vi "ActiView806-Lores.vi"() -> ()   [LabVIEW 2020] (continued)
                  n1614 = call "DCviewer-Mon.vi"("N Chan In"=w4217, "Speedmode"=w4199, "Mark2"=w4201, "Channels"="Offset", "ElecGain"=w4213) -> ("First Trace"=w4218:i32, "First Half array out"=→"Offset Graph First Half":dbl[], "First Half Graph Scaling"=w4212:T36, "Second Half array out"=→"Offset Graph  Second Half":dbl[], "Second Half Graph Scaling"=w4220:T36)
                  n1615 = property on="Offset Graph First Half" class="WFGraph (strict)"() -> ("Position:Left"=w4230:i32)  [unwired: 2 in, 2 out]
                  n1616 = call "DCviewer-TP.vi"("ElecGain"=w4213, "Mark2"=w4201, "Speedmode"=w4199, "N Chan In"=w4217) -> ("Second Half array out"=→"TP Offset Graph 2":dbl[], "First Half array out"=→"TP Offset Graph 1":dbl[])
                  n1617 = Select(t=u32 16711680, s=w4228, f=u32 1970943) -> (s? t:f=w4203:u32)
                  n1618 = Unbundle(w4212) -> ("Xo"=w4222:dbl, "Xmax"=w4208:dbl, "Xmin"=w4207:dbl, "Marker values"=w4206:dbl[])
                  n1619 = Greater?(x=w4229, y=w4230) -> (0:w4231:bool)
                  n1620 = Negate(x=w4205) -> (-x=w4204:dbl)
                  n1621 = property on="Offset Graph First Half" class="WFGraph (strict)"("Plot.Fill/Pt. Color"=w4203, "X Scale.Offset and Multiplier:Offset"=w4222, "XScale.Maximum"=w4208, "XScale.Minimum"=w4207, "XScale.MarkerVals[]"=w4206) -> ()  [unwired: 2 in, 2 out]
                  n1622 = case shown="False" w4231 {
                    tunnel: w4205 -> [w4317 w4326]
                    tunnel: w4229 -> [w4318 w4325]
                    tunnel: u32 1029 ("Plot Area:Size:Width") -> [w4316 w4324]
                    tunnel: w4204 -> [w4315 w4323]
                    frame False {
                      n1623 = stacked-sequence {
                        tunnel: w4318 -> [w4320 _]
                        tunnel: w4317 -> [_ w4322]
                        tunnel: w4316 -> [w4319 _]
                        tunnel: w4315 -> [_ w4321]
                        frame #0 {
                          n1624 = property on="Offset Graph  Second Half" class="WFGraph (strict)"("Position:Left"=w4320, "Width"=w4319) -> ()  [unwired: 2 in, 2 out]
                          n1625 = property on="Offset Graph First Half" class="WFGraph (strict)"("Position:Left"=w4320, "Width"=w4319) -> ()  [unwired: 2 in, 2 out]
                        }
                        frame #1 {
                          n1626 = property on="Offset Graph First Half" class="WFGraph (strict)"("Y Scale.Range:Maximum"=w4322, "YScale.Minimum"=w4321) -> ()  [unwired: 2 in, 2 out]
                          n1627 = property on="Offset Graph  Second Half" class="WFGraph (strict)"("Y Scale.Range:Maximum"=w4322, "YScale.Minimum"=w4321) -> ()  [unwired: 2 in, 2 out]
                        }
                      }
                    }
                    frame True {
                      n1628 = stacked-sequence {
                        tunnel: w4325 -> [_ w4330]
                        tunnel: w4326 -> [w4328 _]
                        tunnel: w4324 -> [_ w4329]
                        tunnel: w4323 -> [w4327 _]
                        frame #0 {
                          n1629 = property on="Offset Graph First Half" class="WFGraph (strict)"("Y Scale.Range:Maximum"=w4328, "YScale.Minimum"=w4327) -> ()  [unwired: 2 in, 2 out]
                          n1630 = property on="Offset Graph  Second Half" class="WFGraph (strict)"("Y Scale.Range:Maximum"=w4328, "YScale.Minimum"=w4327) -> ()  [unwired: 2 in, 2 out]
                        }
                        frame #1 {
                          n1631 = property on="Offset Graph  Second Half" class="WFGraph (strict)"("Position:Left"=w4330, "Width"=w4329) -> ()  [unwired: 2 in, 2 out]
                          n1632 = property on="Offset Graph First Half" class="WFGraph (strict)"("Position:Left"=w4330, "Width"=w4329) -> ()  [unwired: 2 in, 2 out]
                        }
                      }
                    }
                  }
                  n1633 = Unbundle(w4220) -> ("Xo"=w4221:dbl, "Xmax"=w4211:dbl, "Xmin"=w4210:dbl, "Marker values"=w4209:dbl[])
                  n1634 = call "DClabels.vi"("Offset"="Offset", "Mark2"=w4201, "Speedmode"=w4199, "Mon Channels"=w4200, "Spec Labels"=w4197) -> ("DC Labels"=w4202:string[])
                  n1635 = for {
                    N: w4219 -> [_]
                    tunnel: w4202 -> [w4242]
                    tunnel: w4218 -> [w4235]
                    i -> [w4237]
                    w4245 = 0
                    w4246 = "\r"
                    n1636 = Add(x=w4235, y=w4237) -> (x+y=w4236:i32)
                    n1637 = Index Array(array=w4242, index=w4236) -> (element=w4238:string)
                    n1638 = Increment(x=w4245) -> (x+1=w4241:i32)
                    n1639 = Increment(x=w4241) -> (x+1=w4244:i32)
                    n1640 = Increment(x=w4244) -> (x+1=w4243:i32)
                    n1641 = String Subset(string=w4238, offset (0)=w4244, length (rest)=w4241) -> (substring=w4248:string)
                    n1642 = String Subset(string=w4238, offset (0)=w4245, length (rest)=w4241) -> (substring=w4250:string)
                    n1643 = String Subset(string=w4238, offset (0)=w4241, length (rest)=w4241) -> (substring=w4249:string)
                    n1644 = String Subset(string=w4238, offset (0)=w4243, length (rest)=w4241) -> (substring=w4247:string)
                    n1645 = Increment(x=w4237) -> (x+1=w4239:i32)
                    n1646 = Concatenate Strings(w4250, w4246, w4249, w4246, w4248, w4246, w4247) -> (w4240:string)
                    n1647 = case shown="64, Default" w4239 {
                      tunnel: w4240 -> [w4251 w4252 w4253 w4254 w4255 w4256 w4257 w4258 w4259 w4260 w4261 w4262 w4263 w4264 w4265 w4266 w4267 w4268 w4269 w4270 w4271 w4272 w4273 w4274 w4275 w4276 w4277 w4278 w4279 w4280 w4281 w4282 w4283 w4284 w4285 w4286 w4287 w4288 w4289 w4290 w4291 w4292 w4293 w4294 w4295 w4296 w4297 w4298 w4299 w4300 w4301 w4302 w4303 w4304 w4305 w4306 w4307 w4308 w4309 w4310 w4311 w4312 w4313 w4314]
                      frame 1 {
                        "Offset1" <- w4251
                      }
                      frame 2 {
                        "Offset2" <- w4252
                      }
                      frame 3 {
                        "Offset3" <- w4253
                      }
                      frame 4 {
                        "Offset4" <- w4254
                      }
                      frame 5 {
                        "Offset5" <- w4255
                      }
                      frame 6 {
                        "Offset6" <- w4256
                      }
                      frame 7 {
                        "Offset7" <- w4257
                      }
                      frame 8 {
                        "Offset8" <- w4258
                      }
                      frame 9 {
                        "Offset9" <- w4259
                      }
                      frame 10 {
                        "Offset10" <- w4260
                      }
                      frame 11 {
                        "Offset11" <- w4261
                      }
                      frame 12 {
                        "Offset12" <- w4262
                      }
                      frame 13 {
                        "Offset13" <- w4263
                      }
                      frame 14 {
                        "Offset14" <- w4264
                      }
                      frame 15 {
                        "Offset15" <- w4265
                      }
                      frame 16 {
                        "Offset16" <- w4266
                      }
                      frame 17 {
                        "Offset17" <- w4267
                      }
                      frame 18 {
                        "Offset18" <- w4268
                      }
                      frame 19 {
                        "Offset19" <- w4269
                      }
                      frame 20 {
                        "Offset20" <- w4270
                      }
                      frame 21 {
                        "Offset21" <- w4271
                      }
                      frame 22 {
                        "Offset22" <- w4272
                      }
                      frame 23 {
                        "Offset23" <- w4273
                      }
                      frame 24 {
                        "Offset24" <- w4274
                      }
                      frame 25 {
                        "Offset25" <- w4275
                      }
                      frame 26 {
                        "Offset26" <- w4276
                      }
                      frame 27 {
                        "Offset27" <- w4277
                      }
                      frame 28 {
                        "Offset28" <- w4278
                      }
                      frame 29 {
                        "Offset29" <- w4279
                      }
                      frame 30 {
                        "Offset30" <- w4280
                      }
                      frame 31 {
                        "Offset31" <- w4281
                      }
                      frame 32 {
                        "Offset32" <- w4282
                      }
                      frame 33 {
                        "Offset33" <- w4283
                      }
                      frame 34 {
                        "Offset34" <- w4284
                      }
                      frame 35 {
                        "Offset35" <- w4285
                      }
                      frame 36 {
                        "Offset36" <- w4286
                      }
                      frame 37 {
                        "Offset37" <- w4287
                      }
                      frame 38 {
                        "Offset38" <- w4288
                      }
                      frame 39 {
                        "Offset39" <- w4289
                      }
                      frame 40 {
                        "Offset40" <- w4290
                      }
                      frame 41 {
                        "Offset41" <- w4291
                      }
                      frame 42 {
                        "Offset42" <- w4292
                      }
                      frame 43 {
                        "Offset43" <- w4293
                      }
                      frame 44 {
                        "Offset44" <- w4294
                      }
                      frame 45 {
                        "Offset45" <- w4295
                      }
                      frame 46 {
                        "Offset46" <- w4296
                      }
                      frame 47 {
                        "Offset47" <- w4297
                      }
                      frame 48 {
                        "Offset48" <- w4298
                      }
                      frame 49 {
                        "Offset49" <- w4299
                      }
                      frame 50 {
                        "Offset50" <- w4300
                      }
                      frame 51 {
                        "Offset51" <- w4301
                      }
                      frame 52 {
                        "Offset52" <- w4302
                      }
                      frame 53 {
                        "Offset53" <- w4303
                      }
                      frame 54 {
                        "Offset54" <- w4304
                      }
                      frame 55 {
                        "Offset55" <- w4305
                      }
                      frame 56 {
                        "Offset56" <- w4306
                      }
                      frame 57 {
                        "Offset57" <- w4307
                      }
                      frame 58 {
                        "Offset58" <- w4308
                      }
                      frame 59 {
                        "Offset59" <- w4309
                      }
                      frame 60 {
                        "Offset60" <- w4310
                      }
                      frame 61 {
                        "Offset61" <- w4311
                      }
                      frame 62 {
                        "Offset62" <- w4312
                      }
                      frame 63 {
                        "Offset63" <- w4313
                      }
                      frame 64, Default {
                        "Offset64" <- w4314
                      }
                    }
                  }
                  n1648 = property on="Offset Graph  Second Half" class="WFGraph (strict)"("Plot.Fill/Pt. Color"=w4203, "X Scale.Offset and Multiplier:Offset"=w4221, "XScale.Maximum"=w4211, "XScale.Minimum"=w4210, "XScale.MarkerVals[]"=w4209) -> ()  [unwired: 2 in, 2 out]
                  n1649 = property on="TP Offset Graph 1" class="WFGraph (strict)"("YScale.Maximum"=w4205, "YScale.Minimum"=w4204, "Plot.Fill/Pt. Color"=w4203) -> ()  [unwired: 2 in, 2 out]
                  n1650 = property on="TP Offset Graph 2" class="WFGraph (strict)"("YScale.Maximum"=w4205, "YScale.Minimum"=w4204, "Plot.Fill/Pt. Color"=w4203) -> ()  [unwired: 2 in, 2 out]
                }
                frame "About ActiView", Default {
                }
              }
              n1651 = Add(x=w3354, y=w3417) -> (x+y=w3430:i32)
              n1652 = Concatenate Strings(w3370, " %" ("string")) -> (→"Jazz Batt Perc":string)
              n1653 = case shown="2" w3741 {
                tunnel: [FALSE FALSE TRUE] -> w3404
                tunnel: [i8 0 i8 2 i8 0] -> w3688
                tunnel: [FALSE TRUE FALSE] -> w3650
                frame 0, Default {
                }
                frame 1 {
                }
                frame 2 {
                }
              }
              n1654 = And(x=w3404, y="AuxReset") -> (x .and. y?=w3678:bool)
              n1655 = Or(x=w3678, y=w3681) -> (x .or. y?=w3680:bool)
              n1656 = call "Sensor.vi"("First Call"=w3431, "BreathBelt"=w3346, "Gain Cluster"=w3642, "Reset Traces"=w3680, "Sample Rate"=w3416, "Sensor Selection"="AuxFree", "8 Channel Aux Array In"=w3677) -> ("Battery Voltage"=w3548:u8, "Temperature"=→"Degrees Celcius":dbl, "Chart Array"=w3606:dbl[][], "GSR2"=→"GSR2":dbl, "GSR1"=→"GSR1":dbl)
              n1657 = Select(t=w3548, s=w3671, f=u8 0 ("t")) -> (s? t:f=→"Battery\nCapacitance" →"Battery":u8)
              n1658 = call "DeciScreen.vi"("Decimating factor"=w3401, "uV/div"=w3607, "Screen Array In"=w3606, "Max Nr of Traces"=w3550) -> ("Chart Array Out"=→"Aux Chart":dbl[][])
              n1659 = And(x=w3419, y=w3522) -> (x .and. y?=w3661:bool)
              n1660 = Unbundle By Name(w3377) -> ("Sync Errors"=w3378:i16, "Recent Sync Error"=w3374:bool)
              n1661 = Add(x="BipFree", y=w3388) -> (x+y=w3414:i32[])
              n1662 = Add(x="AnaFree", y=w3430) -> (x+y=w3410:i32[])
              n1663 = And(x="AnaReset", y=w3404) -> (x .and. y?=w3567:bool)
              n1664 = Bundle("AvgLP"="AvgLP", "AvgLPfreq"="AvgLPfreq", "AvgHP"="AvgHP", "AvgHPfreq"="AvgHPfreq") -> (w3620:T37)  [unwired: 1 out]
              n1665 = call "Ref-Avg-New.vi"("MonFreeAvg1"="MonFreeAvg1", "N Channel Array In"=w3405, "RefFreeAvg1"="RefFreeAvg1", "MonFreeAvg2"="MonFreeAvg2", "Sample Rate"=w3416, "RefFreeAvg2"="RefFreeAvg2", "Initialize Filters"=w3431, "HP Cluster"=w3620) -> ("2 Avg Chan Out"=w3610:dbl[][])
              n1666 = Not(x=w3356) -> (.not. x?=w3360:bool)
              n1667 = Less Or Equal?(x=w3357, y=u8 5) -> (x <= y?=w3359:bool)
              n1668 = Equal To 0?(x="TrigCode") -> (x = 0?=w3500:bool)
              n1669 = Compound Arithmetic op=AND(w3360, w3359, w3353) -> (w3358:bool)
              n1670 = Not Equal To 0?(x=w3354) -> (x != 0?=w3428:bool)
              n1671 = Not Equal To 0?(x=w3415) -> (x != 0?=w3382:bool)
              n1672 = Not Equal To 0?(x=w3413) -> (x != 0?=w3517:bool)
              n1673 = Array Size(array=w3610) -> (size(s)=w3627:i32[])
              n1674 = Add(x=w3378, y=w3379) -> (x+y=w3376:i16)
              "Errors:" <- w3376
              n1675 = Not Equal To 0?(x=w3379) -> (x != 0?=w3373:bool)
              n1676 = case shown="14" "Channels" {
                tunnel: [i32[] [0, 1, 2, 3, 4, 5, 6, 7, 8, 9, 10, 11, 12, 13, 14, 15, 16, 17, 18, 19, 20, 21, 22, 23, 24, 25, 26, 27, 28, 29, 30, 31, 32, 33, 34, 35, 36, 37, 38, 39, 40, 41, 42, 43, 44, 45, 46, 47, 48, 49, 50, 51, 52, 53, 54, 55, 56, 57, 58, 59, 60, 61, 62, 63, 64, 65, 66, 67, 68, 69, 70, 71, 72, 73, 74, 75, 76, 77, 78, 79, 80, 81, 82, 83, 84, 85, 86, 87, 88, 89, 90, 91, 92, 93, 94, 95, 96, 97, 98, 99, 100, 101, 102, 103, 104, 105, 106, 107, 108, 109, 110, 111, 112, 113, 114, 115, 116, 117, 118, 119, 120, 121, 122, 123, 124, 125, 126, 127, 128, 129, 130, 131, 132, 133, 134, 135, 136, 137, 138, 139, 140, 141, 142, 143, 144, 145, 146, 147, 148, 149, 150, 151, 152, 153, 154, 155, 156, 157, 158, 159, 160, 161, 162, 163, 164, 165, 166, 167, 168, 169, 170, 171, 172, 173, 174, 175, 176, 177, 178, 179, 180, 181, 182, 183, 184, 185, 186, 187, 188, 189, 190, 191, 192, 193, 194, 195, 196, 197, 198, 199, 200, 201, 202, 203, 204, 205, 206, 207, 208, 209, 210, 211, 212, 213, 214, 215, 216, 217, 218, 219, 220, 221, 222, 223, 224, 225, 226, 227, 228, 229, 230, 231, 232, 233, 234, 235, 236, 237, 238, 239, 240, 241, 242, 243, 244, 245, 246, 247, 248, 249, 250, 251, 252, 253, 254, 255, 256, 257, 258, 259, 260, 261, 262, 263] ("Array") i32[] [0, 1, 2, 3, 4, 5, 6, 7, 8, 9, 10, 11, 12, 13, 14, 15, 16, 17, 18, 19, 20, 21, 22, 23, 24, 25, 26, 27, 28, 29, 30, 31, 32, 33, 34, 35, 36, 37, 38, 39, 40, 41, 42, 43, 44, 45, 46, 47, 48, 49, 50, 51, 52, 53, 54, 55, 56, 57, 58, 59, 60, 61, 62, 63, 64, 65, 66, 67, 68, 69, 70, 71, 72, 73, 74, 75, 76, 77, 78, 79, 80, 81, 82, 83, 84, 85, 86, 87, 88, 89, 90, 91, 92, 93, 94, 95, 96, 97, 98, 99, 100, 101, 102, 103, 104, 105, 106, 107, 108, 109, 110, 111, 112, 113, 114, 115, 116, 117, 118, 119, 120, 121, 122, 123, 124, 125, 126, 127, 128, 129, 130, 131, 132, 133, 134, 135, 136, 137, 138, 139, 140, 141, 142, 143, 144, 145, 146, 147, 148, 149, 150, 151, 152, 153, 154, 155, 156, 157, 158, 159, 160, 161, 162, 163, 164, 165, 166, 167, 168, 169, 170, 171, 172, 173, 174, 175, 176, 177, 178, 179, 180, 181, 182, 183, 184, 185, 186, 187, 188, 189, 190, 191, 192, 193, 194, 195, 196, 197, 198, 199, 200, 201, 202, 203, 204, 205, 206, 207, 208, 209, 210, 211, 212, 213, 214, 215, 216, 217, 218, 219, 220, 221, 222, 223, 224, 225, 226, 227, 228, 229, 230, 231, 232, 233, 234, 235, 236, 237, 238, 239, 240, 241, 242, 243, 244, 245, 246, 247, 248, 249, 250, 251, 252, 253, 254, 255] ("All Channels") i32[] [0, 1, 2, 3, 4, 5, 6, 7, 8, 9, 10, 11, 12, 13, 14, 15, 16, 17, 18, 19, 20, 21, 22, 23, 24, 25, 26, 27, 28, 29, 30, 31, 32, 33, 34, 35, 36, 37, 38, 39, 40, 41, 42, 43, 44, 45, 46, 47, 48, 49, 50, 51, 52, 53, 54, 55, 56, 57, 58, 59, 60, 61, 62, 63, 64, 65, 66, 67, 68, 69, 70, 71, 72, 73, 74, 75, 76, 77, 78, 79, 80, 81, 82, 83, 84, 85, 86, 87, 88, 89, 90, 91, 92, 93, 94, 95, 96, 97, 98, 99, 100, 101, 102, 103, 104, 105, 106, 107, 108, 109, 110, 111, 112, 113, 114, 115, 116, 117, 118, 119, 120, 121, 122, 123, 124, 125, 126, 127, 128, 129, 130, 131, 132, 133, 134, 135, 136, 137, 138, 139, 140, 141, 142, 143, 144, 145, 146, 147, 148, 149, 150, 151, 152, 153, 154, 155, 156, 157, 158, 159] ("Array") i32[] [0, 1, 2, 3, 4, 5, 6, 7, 8, 9, 10, 11, 12, 13, 14, 15, 16, 17, 18, 19, 20, 21, 22, 23, 24, 25, 26, 27, 28, 29, 30, 31, 32, 33, 34, 35, 36, 37, 38, 39, 40, 41, 42, 43, 44, 45, 46, 47, 48, 49, 50, 51, 52, 53, 54, 55, 56, 57, 58, 59, 60, 61, 62, 63, 64, 65, 66, 67, 68, 69, 70, 71, 72, 73, 74, 75, 76, 77, 78, 79, 80, 81, 82, 83, 84, 85, 86, 87, 88, 89, 90, 91, 92, 93, 94, 95, 96, 97, 98, 99, 100, 101, 102, 103, 104, 105, 106, 107, 108, 109, 110, 111, 112, 113, 114, 115, 116, 117, 118, 119, 120, 121, 122, 123, 124, 125, 126, 127] ("Array") i32[] [0, 1, 2, 3, 4, 5, 6, 7, 8, 9, 10, 11, 12, 13, 14, 15, 16, 17, 18, 19, 20, 21, 22, 23, 24, 25, 26, 27, 28, 29, 30, 31, 32, 33, 34, 35, 36, 37, 38, 39, 40, 41, 42, 43, 44, 45, 46, 47, 48, 49, 50, 51, 52, 53, 54, 55, 56, 57, 58, 59, 60, 61, 62, 63] ("Array") i32[] [0, 1, 2, 3, 4, 5, 6, 7, 8, 9, 10, 11, 12, 13, 14, 15, 16, 17, 18, 19, 20, 21, 22, 23, 24, 25, 26, 27, 28, 29, 30, 31] ("Array") i32[] [32, 33, 34, 35, 36, 37, 38, 39, 40, 41, 42, 43, 44, 45, 46, 47, 48, 49, 50, 51, 52, 53, 54, 55, 56, 57, 58, 59, 60, 61, 62, 63] ("Array") i32[] [64, 65, 66, 67, 68, 69, 70, 71, 72, 73, 74, 75, 76, 77, 78, 79, 80, 81, 82, 83, 84, 85, 86, 87, 88, 89, 90, 91, 92, 93, 94, 95] ("Array") i32[] [96, 97, 98, 99, 100, 101, 102, 103, 104, 105, 106, 107, 108, 109, 110, 111, 112, 113, 114, 115, 116, 117, 118, 119, 120, 121, 122, 123, 124, 125, 126, 127] ("Array") i32[] [128, 129, 130, 131, 132, 133, 134, 135, 136, 137, 138, 139, 140, 141, 142, 143, 144, 145, 146, 147, 148, 149, 150, 151, 152, 153, 154, 155, 156, 157, 158, 159] ("Array") i32[] [160, 161, 162, 163, 164, 165, 166, 167, 168, 169, 170, 171, 172, 173, 174, 175, 176, 177, 178, 179, 180, 181, 182, 183, 184, 185, 186, 187, 188, 189, 190, 191] ("Array") i32[] [192, 193, 194, 195, 196, 197, 198, 199, 200, 201, 202, 203, 204, 205, 206, 207, 208, 209, 210, 211, 212, 213, 214, 215, 216, 217, 218, 219, 220, 221, 222, 223] ("Array") i32[] [224, 225, 226, 227, 228, 229, 230, 231, 232, 233, 234, 235, 236, 237, 238, 239, 240, 241, 242, 243, 244, 245, 246, 247, 248, 249, 250, 251, 252, 253, 254, 255] ("Array") w4472 w4475] -> w3389
                tunnel: [w4444 w4446 w4448 w4450 w4452 w4454 w4456 w4458 w4460 w4462 w4464 w4466 w4468 w4470 T5."Enabled" ("Disabled")] -> w3390
                tunnel: w3388 -> [_ _ _ _ _ _ _ _ _ _ _ _ _ w4471 _]
                tunnel: "MonFree" -> [_ _ _ _ _ _ _ _ _ _ _ _ _ _ w4475]
                tunnel: T5."Disabled and Grayed Out" ("Disabled") -> [w4444 w4446 w4448 w4450 w4452 w4454 w4456 w4458 w4460 w4462 w4464 w4466 w4468 w4470 _]
                frame 0, Default {
                }
                frame 1 {
                }
                frame 2 {
                }
                frame 3 {
                }
                frame 4 {
                }
                frame 5 {
                }
                frame 6 {
                }
                frame 7 {
                }
                frame 8 {
                }
                frame 9 {
                }
                frame 10 {
                }
                frame 11 {
                }
                frame 12 {
                }
                frame 13 {
                  n1677 = Add(x=i32[] [0, 1, 2, 3, 4, 5, 6, 7] ("Array"), y=w4471) -> (x+y=w4472:i32[])
                }
                frame 14 {
                }
              }
              n1678 = Add(x="JazzFree", y=w3417) -> (x+y=w3402:i32[])
              n1679 = Not(x=w3500) -> (.not. x?=w3639:bool)
              n1680 = Select(t=w3410, s=w3517, f=i32[] []) -> (s? t:f=w3518:i32[])
              n1681 = And(x="JazzReset", y=w3404) -> (x .and. y?=w3423:bool)
              n1682 = Select(t=w3402, s=w3428, f=i32[] []) -> (s? t:f=w3424:i32[])
              n1683 = Index Array(array=w3627) -> (element=w3622:i32)  [unwired: 1 in]
              n1684 = case shown="True" w3631 {
                selector: w3631 -> [_ w3951]
                tunnel: w3636 -> [w3948 _]
                tunnel: w3637 -> [w3949 _]
                tunnel: [w3949 w3962] -> w3400
                tunnel: [w3948 w3962] -> w3399
                tunnel: w3622 -> [_ w3961]
                tunnel: w3629 -> [w3947 w3950]
                tunnel: [w3947 w3960] -> w3630
                tunnel: w3459 -> [_ w3955]
                frame False {
                }
                frame True {
                  w3952 = 0 ("Rejected Sweeps")
                  # "Initilaize Buffers"
                  n1685 = Multiply(x="AvgSweep", y=w3955) -> (x*y=w3959:i32)
                  n1686 = To Double Precision Float(number=w3959) -> (double precision float=w3958:dbl)
                  n1687 = Divide(x=w3958, y=1000.0) -> (x/y=w3956:dbl)
                  n1688 = To Long Integer(number=w3956) -> (32bit integer=w3953:i32)
                  n1689 = local write "Valid Sweeps"(w3952) -> ()
                  n1690 = Bundle By Name(cluster=w3950, "Start Averaging"=w3951, "Busy Averaging"=w3951, "Sweep Lenght in Samples"=w3953, "Valid Sweeps"=w3952, "Rejected Sweeps"=w3952, "First Graph Update"=w3951) -> (w3960:T11)
                  n1691 = Initialize Array(0.0 ("element"), w3961, w3953) -> (w3962:dbl[][])
                  n1692 = local write "Rejected Sweeps"(w3952) -> ()
                }
              }
              n1693 = Select(t=w3414, s=w3382, f=i32[] []) -> (s? t:f=w3525:i32[])
              n1694 = And(x=w3374, y=w3373) -> (x .and. y?=w3453:bool)
              n1695 = property on="Trigger Code" class="Pict"("Visible"=w3639) -> ()  [unwired: 2 in, 2 out]
              n1696 = call "Ref-Jazz1.vi"("Initialize Filters"=w3425, "Center Traces"=w3423, "Channels"=w3424, "Channel Array In"=w3405) -> ("Screen signals Out"=w3447:dbl[][])  [unwired: 4 out]
              n1697 = property on="Trigger Chart" class="WFChart (strict)"("Visible"=w3500) -> ()  [unwired: 2 in, 2 out]
              n1698 = Select(t=T5."Disabled and Grayed Out" ("Disabled"), s=w3403, f=T5."Enabled" ("Disabled")) -> (s? t:f=w3418:T5)
              n1699 = Array Size(array=w3424) -> (size(s)=w3437:i32)
              n1700 = case shown="True" "AddTP" {
                tunnel: w3389 -> [w3755 w3757]
                tunnel: [w3755 w3756] -> w3387
                tunnel: w3388 -> [_ w3759]
                frame False {
                }
                frame True {
                  n1701 = Add(x=i32[] [0, 1, 2, 3, 4, 5, 6, 7] ("Array"), y=w3759) -> (x+y=w3758:i32[])
                  n1702 = Build Array (concatenate)(w3757, w3758) -> (w3756:i32[])
                }
              }
              n1703 = Array Size(array=w3442) -> (size(s)=w3444:i32)
              n1704 = property on="JazzFree" class="LstBox (strict)"("Disabled"=w3418) -> ()  [unwired: 2 in, 2 out]
              n1705 = Not Equal?(x=w3437, y=w3444) -> (x != y?=w3432:bool)
              n1706 = Not Equal?(x=w3424, y=w3442) -> (x != y?=w3443:bool[])
              n1707 = property on="Dummy String" class="Str"("Visible"=w3500) -> ()  [unwired: 2 in, 2 out]
              n1708 = Bundle("MonLP"="MonLP", "MonLPfreq"="MonLPfreq", "MonHP"="MonHP", "MonHPfreq"="MonHPfreq") -> (w3719:T38)  [unwired: 1 out]
              n1709 = Or Array Elements(Boolean array=w3443) -> (logical OR=w3434:bool)
              n1710 = Bundle("BipLP"="BipLP", "BipLPfreq"="BipLPfreq", "BipHP"="BipHP", "BipHPfreq"="BipHPfreq") -> (w3597:T39)  [unwired: 1 out]
              n1711 = call "Ref-Bip-New.vi"("Channel Array In"=w3405, "Channels"=w3525, "Center Traces"=w3404, "Initialize Filter"=w3683, "Sample Rate"=w3416, "Filter Cluster"=w3597, "ElecGain"=w3348) -> ("Screen signals Out"=w3682:dbl[][])
              n1712 = Bundle By Name(cluster=w3377, "Sync Errors"=w3376, "Recent Sync Error"=w3373) -> (w3375:T27)
              n1713 = Bundle("AnaLP"="AnaLP", "AnaLPfreq"="AnaLPfreq", "AnaHP"="AnaHP", "AnaHPfreq"="AnaHPfreq") -> (w3647:T40)  [unwired: 1 out]
              n1714 = call "Ref-Ana.vi"("Channel Array In"=w3405, "Channels"=w3518, "Center Traces"=w3567, "Initialize Filters"=w3568, "Sample Rate"=w3416, "Filter Cluster"=w3647) -> ("Screen signals Out"=w3649:dbl[][])  [unwired: 1 out]
              n1715 = call "DeciScreen.vi"("Decimating factor"=w3401, "uV/div"=w3426, "Screen Array In"=w3447, "Max Nr of Traces"=w3354) -> ("Chart Array Out"=→"Jazz Chart":dbl[][])
              n1716 = Equal?(x=T2."Analog Input Box" ("Charts/Graphs"), y="Charts/Graphs") -> (x = y?=w3644:bool)
              n1717 = Compound Arithmetic op=OR(w3434, w3432, w3431) -> (w3433:bool)
              n1718 = Array Subset(array=w3387, length=w3381) -> (w3386:i32[])  [unwired: 1 in]
              n1719 = Bundle("Speed Mode"=w3327, "Save Subset"=w3523, w3386, "Add Touchproofs"=w3527, "Mon Channels"=w3388, "Bip Channels"=w3415, "Add Sensors"=w3420, w3411, "Add Jazz"=w3421, w3402, "Add Anas"=w3429, w3410, "Save Box"=w3409) -> (w3529:T41)  [unwired: 1 out]
              n1720 = call "Act_Save_Daisy.vi"("Save Selection Cluster"=w3529, "Status Channel  In"=w3406, "Data In"=w3412, "Samples per Record"=w3459, "BDF Buffer In"=w3458, "Index in Byte In"=w3457) -> ("Nr of Chan Saved"=w3611:i32, "BDF Buffer Out"=w3698:u8[], "Index in Byte Out"=w3699:i32)
              n1721 = Decrement(x=w3611) -> (x-1=w3618:i32)
              n1722 = Format Into String(format string="%d" ("Format String"), w3618) -> (resulting string=w3616:string)  [unwired: 2 in, 1 out]
              n1723 = Concatenate Strings(w3616, " + 1" ("Substring")) -> (w3614:string)
              n1724 = Select(t=w3614, s=w3419, f="0 + 0") -> (s? t:f=→"Nr Chan Saved":string)
              n1725 = Select(t=w3332, s=w3661, f=w3390) -> (s? t:f=w3708:T5)
              n1726 = Select(t=w3332, s=w3661, f=T5."Enabled" ("Disabled")) -> (s? t:f=w3384:T5)
              n1727 = property on="MonFree" class="LstBox (strict)"("Disabled"=w3708) -> ()  [unwired: 2 in, 2 out]
              n1728 = Select(t=w3384, s=w3382, f=w3332) -> (s? t:f=w3383:T5)
              n1729 = property on="Channels" class="Ring (strict)"("Disabled"=w3384) -> ()  [unwired: 2 in, 2 out]
              n1730 = property on="AddTP" class="Bool (strict)"("Disabled"=w3383) -> ()  [unwired: 2 in, 2 out]
              n1731 = case shown="True" w3644 {
                tunnel: w3405 -> [_ w3968]
                tunnel: w3430 -> [_ w3966]
                frame False {
                }
                frame True {
                  n1732 = Add(x=w3966, y="AnaOffset") -> (x+y=w3964:i32)
                  n1733 = call "DCviewer-Ana.vi"("Ana Channels"=w3964, "N Chan In"=w3968) -> ("1 Chan array out"=→"Ana Offset Graph":dbl[])
                }
              }
              n1734 = Unbundle By Name(w3733) -> ("End of Screen"=w3669:bool, "Prop Screen Minimum"=w3665:i64, "Screen Position"=w3504:i32)
              n1735 = call "TriggerScreen.vi"("Screen Position"=w3504, "Downsample Correction"=w3449, "Block Cluster"=w3499, "[user-specified font]"=T13 {"Font Name:"="Microsoft Sans Serif", "Size"=12, "Strikeout?"=FALSE, "Italic?"=FALSE, "Underline?"=FALSE, "Outline?"=FALSE, "Shadow?"=FALSE, "Bold?"=FALSE}, "Old picture 2"=w3407, "Old picture 1"=w3408, "Status Channel  In"=w3406, "TrigCode"="TrigCode") -> ("New picture 2"=w3502:picture, "New picture 1"=w3503:picture)
              n1736 = case shown="\"Auxiliary Sensors\"" "Charts/Graphs" {
                tunnel: [T1."Monopolar" ("Left Sidebar") T1."Bipolar" ("Left Sidebar") T1."Offset" ("Left Sidebar") T1."Average" ("Left Sidebar") T1."Sensors" ("Left Sidebar") T1."Jazz" ("Left Sidebar") T1."Analog" ("Left Sidebar") T1."Initialization" ("Left Sidebar")] -> w3452
                frame "Monopolar Display" {
                }
                frame "Bipolar Leads" {
                }
                frame "Electrode Offset" {
                }
                frame "Event Related Average" {
                }
                frame "Auxiliary Sensors" {
                }
                frame "Jazz Eyetracker" {
                }
                frame "Analog Input Box" {
                }
                frame "About ActiView", Default {
                }
              }
              "Left Sidebar" <- w3452
              n1737 = Select(t=w3503, s=w3542, f=w3502) -> (s? t:f=→"Trigger Code":picture)
              n1738 = case shown="15" "MonScale" {
                tunnel: [5.0 10.0 20.0 50.0 100.0 200.0 500.0 1000.0 2000.0 5000.0 10000.0 20000.0 50000.0 100000.0 200000.0 500000.0] -> w3711
                frame 0, Default {
                }
                frame 1 {
                }
                frame 2 {
                }
                frame 3 {
                }
                frame 4 {
                }
                frame 5 {
                }
                frame 6 {
                }
                frame 7 {
                }
                frame 8 {
                }
                frame 9 {
                }
                frame 10 {
                }
                frame 11 {
                }
                frame 12 {
                }
                frame 13 {
                }
                frame 14 {
                }
                frame 15 {
                }
              }
              n1739 = case shown="18" "AnaScale" {
                tunnel: [5.0 10.0 20.0 50.0 100.0 200.0 500.0 1000.0 2000.0 5000.0 10000.0 20000.0 50000.0 100000.0 200000.0 500000.0 1000000.0 2000000.0 4000000.0] -> w3658
                frame 0, Default {
                }
                frame 1 {
                }
                frame 2 {
                }
                frame 3 {
                }
                frame 4 {
                }
                frame 5 {
                }
                frame 6 {
                }
                frame 7 {
                }
                frame 8 {
                }
                frame 9 {
                }
                frame 10 {
                }
                frame 11 {
                }
                frame 12 {
                }
                frame 13 {
                }
                frame 14 {
                }
                frame 15 {
                }
                frame 16 {
                }
                frame 17 {
                }
                frame 18 {
                }
              }
              n1740 = case shown="15" "BipScale" {
                tunnel: [5.0 10.0 20.0 50.0 100.0 200.0 500.0 1000.0 2000.0 5000.0 10000.0 20000.0 50000.0 100000.0 200000.0 500000.0] -> w3700
                frame 0, Default {
                }
                frame 1 {
                }
                frame 2 {
                }
                frame 3 {
                }
                frame 4 {
                }
                frame 5 {
                }
                frame 6 {
                }
                frame 7 {
                }
                frame 8 {
                }
                frame 9 {
                }
                frame 10 {
                }
                frame 11 {
                }
                frame 12 {
                }
                frame 13 {
                }
                frame 14 {
                }
                frame 15 {
                }
              }
              n1741 = Build Array(w3456, w3455, w3453, w3456, w3356, w3355) -> (w3663:bool[])
              n1742 = Compound Arithmetic op=OR(w3455, w3453, w3356, w3355) -> (w3454:bool)
              n1743 = Array Size(array=w3386) -> (size(s)=w3495:i32)
              n1744 = Array Size(array=w3715) -> (size(s)=w3730:i32)
              n1745 = case shown="True" w3433 {
                tunnel: w3437 -> [_ w3766]
                tunnel: w3424 -> [_ w3763]
                tunnel: w3448 -> [_ w3761]
                frame False {
                }
                frame True {
                  w3764 = 9  # Nr of Jazz Labels
                  w3771 = -292.0  # Upper Y-value
                  w3773 = 532.0  # Lower Y-value
                  n1746 = Not Equal To 0?(x=w3766) -> (x != 0?=w3767:bool)
                  n1747 = Increment(x=w3766) -> (x+1=w3768:i32)
                  n1748 = Subtract(x=w3773, y=w3771) -> (x-y=w3772:dbl)
                  n1749 = Select(t=w3768, s=w3767, f=2) -> (s? t:f=w3762:i32)
                  n1750 = To Double Precision Float(number=w3762) -> (double precision float=w3765:dbl)
                  n1751 = Divide(x=w3772, y=w3765) -> (x/y=w3770:dbl)
                  n1752 = for {
                    N: w3764 -> [_]
                    tunnel: w3761 -> [w3782]
                    tunnel: w3763 -> [w3779]
                    tunnel: w3771 -> [w3784]
                    tunnel: w3770 -> [w3783]
                    tunnel: w3766 -> [w3780]
                    i -> [w3775]
                    n1753 = Greater?(x=w3780, y=w3775) -> (0:w3781:bool)
                    n1754 = Increment(x=w3775) -> (x+1=w3778:i32)
                    n1755 = case shown="True" w3781 {
                      tunnel: w3784 -> [_ w3816]
                      tunnel: w3783 -> [_ w3815]
                      tunnel: w3782 -> [_ w3806]
                      tunnel: w3778 -> [_ w3811]
                      tunnel: ["" w3807] -> w3777
                      tunnel: [0 w3810] -> w3776
                      tunnel: w3779 -> [_ w3809]
                      tunnel: w3775 -> [_ w3808]
                      frame False {
                      }
                      frame True {
                        n1756 = Index Array(array=w3809, index=w3808) -> (element=w3805:i32)
                        n1757 = To Double Precision Float(number=w3811) -> (double precision float=w3814:dbl)
                        n1758 = Index Array(array=w3806, index=w3805) -> (element=w3812:string)
                        n1759 = Multiply(x=w3815, y=w3814) -> (x*y=w3817:dbl)
                        n1760 = Add(x=w3816, y=w3817) -> (x+y=w3818:dbl)
                        n1761 = String Subset(string=w3812, length (rest)=4 ("length (rest)")) -> (substring=w3807:string)  [unwired: 1 out]
                        n1762 = To Long Integer(number=w3818) -> (32bit integer=w3810:i32)
                      }
                    }
                    n1763 = case shown="9, Default" w3778 {
                      tunnel: w3777 -> [w3786 w3788 w3790 w3792 w3794 w3796 w3798 w3800 w3802]
                      tunnel: w3776 -> [w3785 w3787 w3789 w3791 w3793 w3795 w3797 w3799 w3801]
                      frame 1 {
                        n1764 = property on="Jazz1" class="Str"("Top"=w3785) -> ()  [unwired: 2 in, 2 out]
                        "Jazz1" <- w3786
                      }
                      frame 2 {
                        n1765 = property on="Jazz2" class="Str"("Top"=w3787) -> ()  [unwired: 2 in, 2 out]
                        "Jazz2" <- w3788
                      }
                      frame 3 {
                        n1766 = property on="Jazz3" class="Str"("Top"=w3789) -> ()  [unwired: 2 in, 2 out]
                        "Jazz3" <- w3790
                      }
                      frame 4 {
                        n1767 = property on="Jazz4" class="Str"("Top"=w3791) -> ()  [unwired: 2 in, 2 out]
                        "Jazz4" <- w3792
                      }
                      frame 5 {
                        n1768 = property on="Jazz5" class="Str"("Top"=w3793) -> ()  [unwired: 2 in, 2 out]
                        "Jazz5" <- w3794
                      }
                      frame 6 {
                        n1769 = property on="Jazz6" class="Str"("Top"=w3795) -> ()  [unwired: 2 in, 2 out]
                        "Jazz6" <- w3796
                      }
                      frame 7 {
                        n1770 = property on="Jazz7" class="Str"("Top"=w3797) -> ()  [unwired: 2 in, 2 out]
                        "Jazz7" <- w3798
                      }
                      frame 8 {
                        n1771 = property on="Jazz8" class="Str"("Top"=w3799) -> ()  [unwired: 2 in, 2 out]
                        "Jazz8" <- w3800
                      }
                      frame 9, Default {
                        n1772 = property on="Jazz9" class="Str"("Top"=w3801) -> ()  [unwired: 2 in, 2 out]
                        "Jazz9" <- w3802
                      }
                    }
                  }
                  n1773 = To Double Precision Float(number=w3762) -> (double precision float=w3774:dbl)
                  n1774 = property on="Jazz Chart" class="WFChart (strict)"("YScale.Maximum"=w3774) -> ()  [unwired: 2 in, 2 out]
                }
              }
              n1775 = Boolean Array To Number(Boolean array=w3663) -> (number=w3372:u32)
              n1776 = Bundle("AvgAbsReject"="AvgAbsReject", "AvgRelReject"="AvgRelReject") -> (w3396:cluster{"AvgAbsReject":dbl, "AvgRelReject":dbl})  [unwired: 1 out]
              n1777 = case shown="True" w3628 {
                selector: w3628 -> [w3934 _]
                tunnel: w3630 -> [w3933 w3938]
                tunnel: w3610 -> [_ w3946]
                tunnel: [w3932 w3937] -> w3633
                tunnel: [w3931 w3941] -> w3635
                tunnel: "AvgTrigLog" -> [_ w3945]
                tunnel: "AvgTrigSel" -> [_ w3944]
                tunnel: w3400 -> [w3931 w3943]
                tunnel: w3399 -> [w3930 w3942]
                tunnel: [w3930 w3940] -> w3398
                tunnel: w3351 -> [_ w3939]
                tunnel: w3396 -> [_ w3936]
                tunnel: [T16 {"Sweeping"=FALSE, "RejAbs"=FALSE, "RejDif"=FALSE} ("Sweep/Reject Cluster Out") w3935] -> w3394
                frame False {
                  n1778 = Bundle By Name(cluster=w3933, "Busy Averaging"=w3934) -> (w3932:T11)
                }
                frame True {
                  n1779 = call "Avg-Sweep-Rev.vi"("Triggers Boolean"=w3939, "Reject Cluster In"=w3936, "AvgTrigLog"=w3945, "AvgTrigSel"=w3944, "Noise Total"=w3942, "Average Total"=w3943, "Processed signals In"=w3946, "Avg Cluster In"=w3938) -> ("Noise Total Out"=w3940:dbl[][], "Average Total Out"=w3941:dbl[][], "Avg Cluster Out"=w3937:T11, "Sweep/Reject Cluster Out"=w3935:T16)
                }
              }
              n1780 = Not Equal?(x=w3495, y=w3730) -> (x != y?=w3693:bool)
              n1781 = Not Equal?(x=w3386, y=w3715) -> (x != y?=w3729:bool[])
              n1782 = case shown="8" "Reference" {
                tunnel: [i32[] [] i32[] [0, 1, 2, 3, 4, 5, 6, 7, 8, 9, 10, 11, 12, 13, 14, 15, 16, 17, 18, 19, 20, 21, 22, 23, 24, 25, 26, 27, 28, 29, 30, 31, 32, 33, 34, 35, 36, 37, 38, 39, 40, 41, 42, 43, 44, 45, 46, 47, 48, 49, 50, 51, 52, 53, 54, 55, 56, 57, 58, 59, 60, 61, 62, 63, 64, 65, 66, 67, 68, 69, 70, 71, 72, 73, 74, 75, 76, 77, 78, 79, 80, 81, 82, 83, 84, 85, 86, 87, 88, 89, 90, 91, 92, 93, 94, 95, 96, 97, 98, 99, 100, 101, 102, 103, 104, 105, 106, 107, 108, 109, 110, 111, 112, 113, 114, 115, 116, 117, 118, 119, 120, 121, 122, 123, 124, 125, 126, 127, 128, 129, 130, 131, 132, 133, 134, 135, 136, 137, 138, 139, 140, 141, 142, 143, 144, 145, 146, 147, 148, 149, 150, 151, 152, 153, 154, 155, 156, 157, 158, 159, 160, 161, 162, 163, 164, 165, 166, 167, 168, 169, 170, 171, 172, 173, 174, 175, 176, 177, 178, 179, 180, 181, 182, 183, 184, 185, 186, 187, 188, 189, 190, 191, 192, 193, 194, 195, 196, 197, 198, 199, 200, 201, 202, 203, 204, 205, 206, 207, 208, 209, 210, 211, 212, 213, 214, 215, 216, 217, 218, 219, 220, 221, 222, 223, 224, 225, 226, 227, 228, 229, 230, 231, 232, 233, 234, 235, 236, 237, 238, 239, 240, 241, 242, 243, 244, 245, 246, 247, 248, 249, 250, 251, 252, 253, 254, 255, 256, 257, 258, 259, 260, 261, 262, 263] ("Array") i32[] [0, 1, 2, 3, 4, 5, 6, 7, 8, 9, 10, 11, 12, 13, 14, 15, 16, 17, 18, 19, 20, 21, 22, 23, 24, 25, 26, 27, 28, 29, 30, 31, 32, 33, 34, 35, 36, 37, 38, 39, 40, 41, 42, 43, 44, 45, 46, 47, 48, 49, 50, 51, 52, 53, 54, 55, 56, 57, 58, 59, 60, 61, 62, 63, 64, 65, 66, 67, 68, 69, 70, 71, 72, 73, 74, 75, 76, 77, 78, 79, 80, 81, 82, 83, 84, 85, 86, 87, 88, 89, 90, 91, 92, 93, 94, 95, 96, 97, 98, 99, 100, 101, 102, 103, 104, 105, 106, 107, 108, 109, 110, 111, 112, 113, 114, 115, 116, 117, 118, 119, 120, 121, 122, 123, 124, 125, 126, 127, 128, 129, 130, 131, 132, 133, 134, 135, 136, 137, 138, 139, 140, 141, 142, 143, 144, 145, 146, 147, 148, 149, 150, 151, 152, 153, 154, 155, 156, 157, 158, 159, 160, 161, 162, 163, 164, 165, 166, 167, 168, 169, 170, 171, 172, 173, 174, 175, 176, 177, 178, 179, 180, 181, 182, 183, 184, 185, 186, 187, 188, 189, 190, 191, 192, 193, 194, 195, 196, 197, 198, 199, 200, 201, 202, 203, 204, 205, 206, 207, 208, 209, 210, 211, 212, 213, 214, 215, 216, 217, 218, 219, 220, 221, 222, 223, 224, 225, 226, 227, 228, 229, 230, 231, 232, 233, 234, 235, 236, 237, 238, 239, 240, 241, 242, 243, 244, 245, 246, 247, 248, 249, 250, 251, 252, 253, 254, 255] ("All Channels") i32[] [0, 1, 2, 3, 4, 5, 6, 7, 8, 9, 10, 11, 12, 13, 14, 15, 16, 17, 18, 19, 20, 21, 22, 23, 24, 25, 26, 27, 28, 29, 30, 31, 32, 33, 34, 35, 36, 37, 38, 39, 40, 41, 42, 43, 44, 45, 46, 47, 48, 49, 50, 51, 52, 53, 54, 55, 56, 57, 58, 59, 60, 61, 62, 63, 64, 65, 66, 67, 68, 69, 70, 71, 72, 73, 74, 75, 76, 77, 78, 79, 80, 81, 82, 83, 84, 85, 86, 87, 88, 89, 90, 91, 92, 93, 94, 95, 96, 97, 98, 99, 100, 101, 102, 103, 104, 105, 106, 107, 108, 109, 110, 111, 112, 113, 114, 115, 116, 117, 118, 119, 120, 121, 122, 123, 124, 125, 126, 127, 128, 129, 130, 131, 132, 133, 134, 135, 136, 137, 138, 139, 140, 141, 142, 143, 144, 145, 146, 147, 148, 149, 150, 151, 152, 153, 154, 155, 156, 157, 158, 159] ("Array") i32[] [0, 1, 2, 3, 4, 5, 6, 7, 8, 9, 10, 11, 12, 13, 14, 15, 16, 17, 18, 19, 20, 21, 22, 23, 24, 25, 26, 27, 28, 29, 30, 31, 32, 33, 34, 35, 36, 37, 38, 39, 40, 41, 42, 43, 44, 45, 46, 47, 48, 49, 50, 51, 52, 53, 54, 55, 56, 57, 58, 59, 60, 61, 62, 63, 64, 65, 66, 67, 68, 69, 70, 71, 72, 73, 74, 75, 76, 77, 78, 79, 80, 81, 82, 83, 84, 85, 86, 87, 88, 89, 90, 91, 92, 93, 94, 95, 96, 97, 98, 99, 100, 101, 102, 103, 104, 105, 106, 107, 108, 109, 110, 111, 112, 113, 114, 115, 116, 117, 118, 119, 120, 121, 122, 123, 124, 125, 126, 127] ("Array") i32[] [0, 1, 2, 3, 4, 5, 6, 7, 8, 9, 10, 11, 12, 13, 14, 15, 16, 17, 18, 19, 20, 21, 22, 23, 24, 25, 26, 27, 28, 29, 30, 31, 32, 33, 34, 35, 36, 37, 38, 39, 40, 41, 42, 43, 44, 45, 46, 47, 48, 49, 50, 51, 52, 53, 54, 55, 56, 57, 58, 59, 60, 61, 62, 63] ("Array") i32[] [0, 1, 2, 3, 4, 5, 6, 7, 8, 9, 10, 11, 12, 13, 14, 15, 16, 17, 18, 19, 20, 21, 22, 23, 24, 25, 26, 27, 28, 29, 30, 31] ("Array") w4441 "RefFree"] -> w3660
                tunnel: [w4426 w4428 w4430 w4432 w4434 w4436 w4438 w4440 T5."Enabled" ("Disabled")] -> w3726
                tunnel: w3386 -> [_ _ _ _ _ _ _ w4441 _]
                tunnel: w3332 -> [w4426 w4428 w4430 w4432 w4434 w4436 w4438 w4440 _]
                frame 0, Default {
                }
                frame 1 {
                }
                frame 2 {
                }
                frame 3 {
                }
                frame 4 {
                }
                frame 5 {
                }
                frame 6 {
                }
                frame 7 {
                }
                frame 8 {
                }
              }
              n1783 = call "Ref-Mon-Jazz.vi"("ElecGain"=w3348, "Reference"=w3660, "Filter Cluster"=w3719, "Sample Rate"=w3416, "Initialize Filters"=w3720, "Center Traces"=w3404, "Channel Selection"=w3386, "N Channel Array In"=w3405) -> ("Screen signals Out"=w3710:dbl[][])
              n1784 = call "DeciScreen.vi"("Decimating factor"=w3401, "uV/div"=w3711, "Screen Array In"=w3710, "Max Nr of Traces"=w3381) -> ("Chart Array Out"=→"Mon Chart":dbl[][])
              n1785 = Select(t=T5."Disabled and Grayed Out" ("Disabled"), s=w3468, f=T5."Enabled" ("Disabled")) -> (s? t:f=w3643:T5)
              n1786 = Or Array Elements(Boolean array=w3729) -> (logical OR=w3694:bool)
              n1787 = call "DeciScreen.vi"("Decimating factor"=w3401, "uV/div"=w3700, "Screen Array In"=w3682, "Max Nr of Traces"=w3415) -> ("Chart Array Out"=→"Bip Chart":dbl[][])
              n1788 = call "DeciScreen.vi"("Decimating factor"=w3401, "uV/div"=w3658, "Screen Array In"=w3649, "Max Nr of Traces"=w3413) -> ("Chart Array Out"=→"Ana Chart":dbl[][])
              n1789 = property on="AnaFree" class="LstBox (strict)"("Disabled"=w3643) -> ()  [unwired: 2 in, 2 out]
              n1790 = Compound Arithmetic op=OR(w3694, w3693, w3431) -> (w3692:bool)
              n1791 = case shown="True" w3692 {
                tunnel: w3495 -> [_ w4498]
                tunnel: w3448 -> [_ w4503]
                tunnel: w3386 -> [_ w4501]
                frame False {
                }
                frame True {
                  w4496 = -292.0  # Upper Y-value
                  w4497 = 532.0  # Lower Y-value
                  w4500 = 64  # Nr of Mon Labels
                  n1792 = Increment(x=w4498) -> (x+1=w4493:i32)
                  n1793 = Increment(x=w4500) -> (x+1=w4499:i32)
                  n1794 = Quotient & Remainder(x=w4498, y=w4499) -> (floor(x/y)=w4495:i32)  [unwired: 1 out]
                  n1795 = To Double Precision Float(number=w4493) -> (double precision float=w4502:dbl)
                  n1796 = Equal To 0?(x=w4495) -> (x = 0?=w4494:bool)
                  n1797 = property on="Mon Chart" class="WFChart (strict)"("YScale.Maximum"=w4502) -> ()  [unwired: 2 in, 2 out]
                  n1798 = for {
                    N: w4500 -> [_]
                    tunnel: w4503 -> [w4512]
                    tunnel: w4501 -> [w4513]
                    tunnel: w4498 -> [w4510]
                    tunnel: w4495 -> [w4505]
                    tunnel: w4493 -> [w4508]
                    tunnel: w4497 -> [w4507]
                    tunnel: w4496 -> [w4506]
                    tunnel: w4494 -> [w4504]
                    i -> [w4511]
                    n1799 = Increment(x=w4511) -> (x+1=w4509:i32)
                    n1800 = case shown="True" w4504 {
                      tunnel: [w4533 w4566] -> w4515
                      tunnel: [w4532 w4565] -> w4514
                      tunnel: w4509 -> [w4531 w4564]
                      tunnel: w4513 -> [w4534 w4563]
                      tunnel: w4511 -> [w4528 w4559]
                      tunnel: w4512 -> [w4535 w4562]
                      tunnel: w4510 -> [w4520 w4560]
                      tunnel: w4508 -> [_ w4555]
                      tunnel: w4507 -> [w4521 w4554]
                      tunnel: w4506 -> [w4522 w4553]
                      tunnel: w4505 -> [w4516 _]
                      frame False {
                        n1801 = Increment(x=w4516) -> (x+1=w4519:i32)
                        n1802 = To Double Precision Float(number=w4519) -> (double precision float=w4524:dbl)
                        n1803 = Increment(x=w4520) -> (x+1=w4523:i32)
                        n1804 = To Double Precision Float(number=w4523) -> (double precision float=w4525:dbl)
                        n1805 = Divide(x=w4525, y=w4524) -> (x/y=w4526:dbl)
                        n1806 = Subtract(x=w4521, y=w4522) -> (x-y=w4530:dbl)
                        n1807 = Multiply(x=w4519, y=w4528) -> (x*y=w4518:i32)
                        n1808 = Quotient & Remainder(x=w4520, y=w4519) -> (floor(x/y)=w4527:i32)  [unwired: 1 out]
                        n1809 = Divide(x=w4530, y=w4526) -> (x/y=w4529:dbl)
                        n1810 = Add(x=w4518, y=w4516) -> (x+y=w4517:i32)
                        n1811 = Greater?(x=w4527, y=w4528) -> (0:w4536:bool)
                        n1812 = case shown="True" w4536 {
                          tunnel: ["" w4540] -> w4533
                          tunnel: [0 w4547] -> w4532
                          tunnel: w4522 -> [_ w4549]
                          tunnel: w4531 -> [_ w4539]
                          tunnel: w4529 -> [_ w4550]
                          tunnel: w4534 -> [_ w4543]
                          tunnel: w4517 -> [_ w4542]
                          tunnel: w4535 -> [_ w4541]
                          frame False {
                          }
                          frame True {
                            n1813 = Index Array(array=w4543, index=w4542) -> (element=w4544:i32)
                            n1814 = To Double Precision Float(number=w4539) -> (double precision float=w4551:dbl)
                            n1815 = Multiply(x=w4550, y=w4551) -> (x*y=w4552:dbl)
                            n1816 = Index Array(array=w4541, index=w4544) -> (element=w4545:string)
                            n1817 = Add(x=w4549, y=w4552) -> (x+y=w4548:dbl)
                            n1818 = String Subset(string=w4545, length (rest)=4 ("length (rest)")) -> (substring=w4540:string)  [unwired: 1 out]
                            n1819 = To Long Integer(number=w4548) -> (32bit integer=w4547:i32)
                          }
                        }
                      }
                      frame True {
                        n1820 = Subtract(x=w4554, y=w4553) -> (x-y=w4557:dbl)
                        n1821 = To Double Precision Float(number=w4555) -> (double precision float=w4558:dbl)
                        n1822 = Greater?(x=w4560, y=w4559) -> (0:w4561:bool)
                        n1823 = Divide(x=w4557, y=w4558) -> (x/y=w4556:dbl)
                        n1824 = case shown="True" w4561 {
                          tunnel: ["" w4569] -> w4566
                          tunnel: [0 w4576] -> w4565
                          tunnel: w4553 -> [_ w4578]
                          tunnel: w4564 -> [_ w4580]
                          tunnel: w4556 -> [_ w4579]
                          tunnel: w4563 -> [_ w4572]
                          tunnel: w4559 -> [_ w4571]
                          tunnel: w4562 -> [_ w4570]
                          frame False {
                          }
                          frame True {
                            n1825 = Index Array(array=w4572, index=w4571) -> (element=w4573:i32)
                            n1826 = To Double Precision Float(number=w4580) -> (double precision float=w4581:dbl)
                            n1827 = Multiply(x=w4579, y=w4581) -> (x*y=w4582:dbl)
                            n1828 = Index Array(array=w4570, index=w4573) -> (element=w4574:string)
                            n1829 = Add(x=w4578, y=w4582) -> (x+y=w4577:dbl)
                            n1830 = String Subset(string=w4574, length (rest)=4 ("length (rest)")) -> (substring=w4569:string)  [unwired: 1 out]
                            n1831 = To Long Integer(number=w4577) -> (32bit integer=w4576:i32)
                          }
                        }
                      }
                    }
                    n1832 = case shown="64, Default" w4509 {
                      tunnel: w4515 -> [w4584 w4586 w4588 w4590 w4592 w4594 w4596 w4598 w4600 w4602 w4604 w4606 w4608 w4610 w4612 w4614 w4616 w4618 w4620 w4622 w4624 w4626 w4628 w4630 w4632 w4634 w4636 w4638 w4640 w4642 w4644 w4646 w4648 w4650 w4652 w4654 w4656 w4658 w4660 w4662 w4664 w4666 w4668 w4670 w4672 w4674 w4676 w4678 w4680 w4682 w4684 w4686 w4688 w4690 w4692 w4694 w4696 w4698 w4700 w4702 w4704 w4706 w4708 w4710]
